vi "toString.vi"(8 "error in (no error)":errorcluster, 11 "SimpleStringMessage in":refnum<class "SimpleStringMessage.lvclass">) -> (0 "error out":errorcluster, 2 "String":string, 3 "SimpleStringMessage out":refnum<class "SimpleStringMessage.lvclass">)   [LabVIEW 2025, in "SimpleStringMessage.lvclass"]
doc: "Format the message to a string"
uses:
  SimpleStringMessage.lvclass
  SimpleStringMessage.lvclass/SimpleStringMessage.ctl
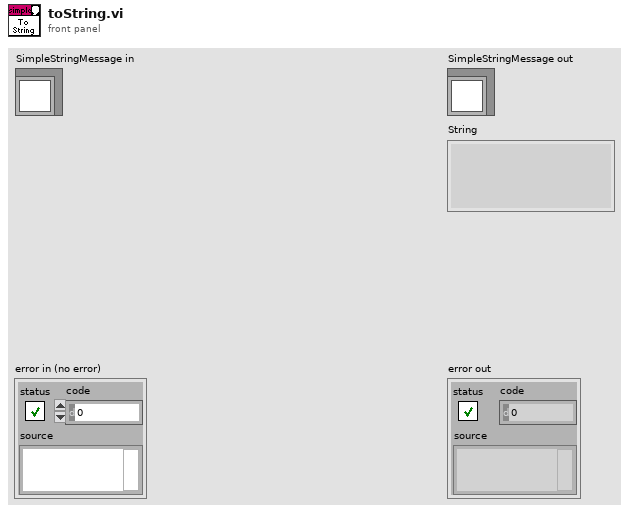
[diagram p1: front panel]
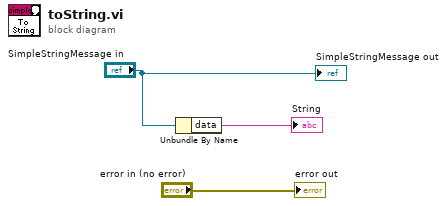
[diagram p0: block diagram]
diagram:
  n1 = Unbundle By Name("SimpleStringMessage in") -> ("data"=→"String":string)
  "error out" <- "error in (no error)"
  "SimpleStringMessage out" <- "SimpleStringMessage in"
